vi "find true.vi"(11 "Array":bool[](array[boolean])) -> (2 "count":u8, 3 "numbers":string)   [LabVIEW 2017, in "SPELS test.lvlib"]
uses:
  SPELS test.lvlib
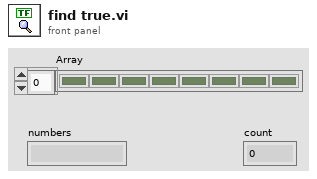
[diagram p1: front panel]
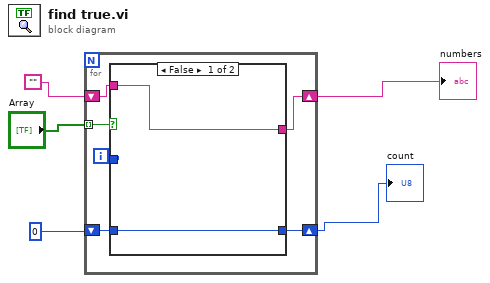
[diagram p0: block diagram]
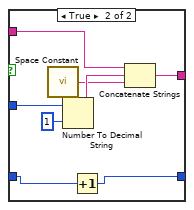
[diagram p2: hidden frame]
diagram:
  n1 = for {
    tunnel: "Array" -> [w11] mode=indexing
    shift-right: [w8] -> w3
    shift-left: "" -> [w10]
    shift-right: [w6] -> w1
    shift-left: u8 0 -> [w7]
    i -> [w9]
    n2 = case shown="False" w11 {
      tunnel: w10 -> [w13 w21]
      tunnel: w9 -> [_ w20]
      tunnel: [w13 w17] -> w8
      tunnel: w7 -> [w12 w15]
      tunnel: [w12 w14] -> w6
      frame False {
      }
      frame True {
        n3 = call <vilib>:"Space Constant.vi"() -> ("String"=w18:string)
        n4 = Number To Decimal String(number=w20, width (-)=i16 1) -> (decimal integer string=w19:string)
        n5 = Increment(x=w15) -> (x+1=w14:u8)
        n6 = Concatenate Strings(w21, w19, w18) -> (w17:string)
      }
    }
  }
  "numbers" <- w3
  "count" <- w1
